vi "ABR3-Create Stimulus.vi"(0 "StimChans":T1[](xcontrol), 1 "Rep In":i32, 9 "Runtime":T26={"Ceiling"=25000.0, "Threshold"=100000.0, "Crossed?"=FALSE, "Step"=0, "Stop"=0, "Avgs"=0, "Level"=0.0, "AI Npts"=0, "Doubled?"=FALSE, "Gain"=0.0, "NWindowPts"=0, "dt"=0.0, "Cal"=path "", "Freq"=0.0, "AO Channels"=[], "AltPol"=FALSE, "AO Npts"=0, "AO Fs"=0.0, "Start"=0, "Stop max"=0, "Ear"=enum."Right", "Waveform"=enum."TONE PIP", "RepRate"=0.0, "CAP or ABR"=1, "LMasker"=0.0, "SeqVar"=enum."Signal Level", "Reps/buffer"=0, "Avg Mode"=enum."Neural/CM", "Wav"=path "", "Order"=enum."Sequential", "Levels"=[], "ControlVal"=0.0, "innerIndex"=0, "indexStep"=0} {"CAP or ABR" items=["CAP", "ABR"]}, 11 "error in (no error)":errorcluster) -> (3 "Rep Out":i32, 4 "StimChans out":T1[](xcontrol), 15 "error out":errorcluster)   [LabVIEW 2020]
uses:
  epl-vi-lib/Signal Synthesis VIs/Controls/Multichannel (Full)/Multichannel (Full).xctl
  TypeDefs/ABR3-Runtime Data.ctl
  epl-vi-lib/Utility VIs/Type Defs/Left-Right ring.ctl
  TypeDefs/ABR-Waveform Enum.ctl
  TypeDefs/ABR3-Seq Var Enum.ctl
  epl-vi-lib/Utility VIs/Array Manipulation VIs/Array-Dimensions (2D).vi
panel:
  out "Elapsed time (ms)":u32
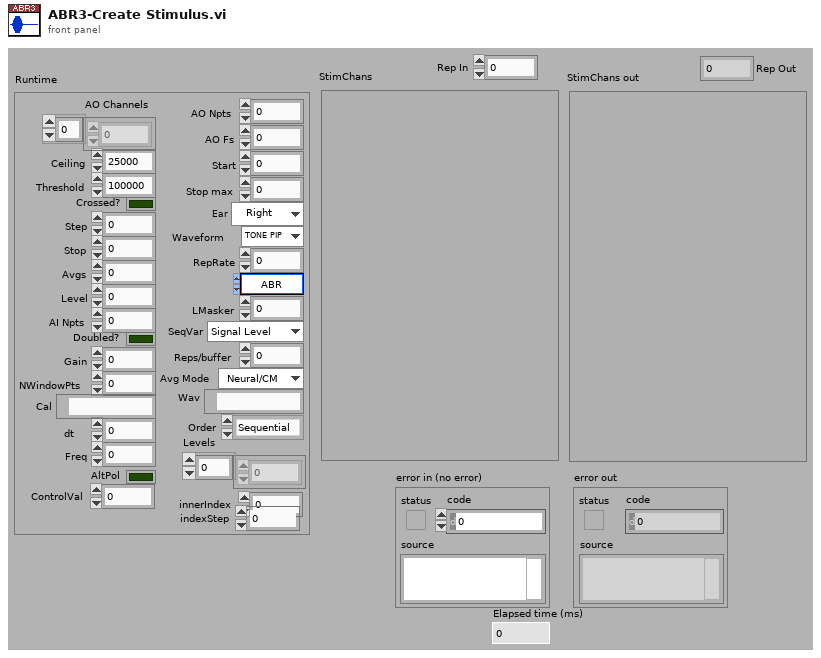
[diagram p1: front panel]
types:
  T1 = typedef "Stimulus Channel (Full).xctl/Full Stimulus Channel Data.ctl" = cluster{"Waveform":T2, "Filter":T19, "Burst":T21, "Level":T22, "Name":string, "Advanced":T24, "SAM":T25}
  T2 = typedef "Waveform XCtl.xctl/Waveform Data.ctl" = cluster{"Type":T3, "Tone":T4, "Pulse Train":T5, "Noise":T8, "File":T9, "FMSweep":T10, "Chirp Train":T11, "Complex Tone":cluster{"Params":T13, "Data":T15}, "Moving Ripple":T16}
  T3 = typedef "Waveform Enum.ctl" = enum16{"OFF", "Tone", "Noise", "Pulse Train", "File", "FM Sweep", "Chirp Train", "Complex Tone", "FM Tone", "Moving Ripple"}
  T4 = typedef "Tone Params.ctl" = cluster{"Frequency (kHz)":dbl, "Last Freq":dbl, "Last Phase":dbl}
  T5 = typedef "Pulse Train Params.ctl" = cluster{"Pulse width (us)":dbl, "Pulse rate (Hz)":dbl, "Gap (ms)":dbl, "Polarity":T6, "PT State":T7, "Asynch":bool}
  T6 = typedef "Pulse Polarity.ctl" = enum16{"POS", "NEG", "POS-NEG", "NEG-POS"}
  T7 = typedef "PT-Continuous State.ctl" = cluster{"Template":dbl[], "Nperiod":i32, "Index":i32, "Pulse Rate (Hz)":dbl, "Phase (cycles)":dbl, "Noff":i32}
  T8 = typedef "Noise Params.ctl" = cluster{"InvFilt":bool, "Noise":dbl[], "CurPt":i32, "Aweight":bool, "Seed":i32, "afile":path}
  T9 = typedef "StimFile-Params.ctl" = cluster{"Filename":path, "Signal":dbl[], "Channel":i32, "stream":bool, "offset":i32, "nreps":i32, "loops":i32, "Randomize":bool, "order":i32[], "Seed":i32, "Tokens":i32}
  T10 = typedef "FM Sweep Params.ctl" = cluster{"Rate (oct/s)":dbl, "Fmin (Hz)":dbl, "Fmax (Hz)":dbl, "Ramp (ms)":dbl, "Linear":bool}
  T11 = typedef "Chirp Train.ctl" = cluster{"Params":T12, "Data":cluster{"WF":dbl[]}}
  T12 = typedef "Chirp Train Params.ctl" = cluster{"Fmin (kHz)":dbl, "Fmax (kHz)":dbl, "Compensate":bool, "Duration (ms)":dbl}
  T13 = typedef "CT-Params.ctl" = cluster{"F0 (Hz)":dbl, "Band":cluster{"Flow (Hz)":dbl, "Fhigh (Hz)":dbl}, "Phase":T14, "Min F0 (Hz)":dbl, "Max F0 (Hz)":dbl, "ContinRandPhase":bool, "Max peak factor":dbl, "Max mod depth":dbl, "MinHarmNum":i32, "MaxHarmNum":i32, "Level Mode":enum16{"per component", "overall rms"}, "% jitter":dbl}
  T14 = typedef "CT-Phase Enum.ctl" = enum16{"Cosine", "Random", "Alternating"}
  T15 = typedef "CT-Runtime Data.ctl" = cluster{"Ncomp":i32, "MinHarm":i32, "Phase":dbl[], "Amplitude":dbl[], "Npts/frame":i32, "Last F0":dbl, "Fmin":dbl, "Fmax":dbl, "Lslope":dbl, "randphase":bool, "overall rms":bool, "fmult":dbl[], "jittered":bool}
  T16 = typedef "Moving Ripple.ctl" = cluster{"Params":T17, "Data":T18}
  T17 = typedef "Moving Ripple.Params.ctl" = cluster{"Fmin":dbl, "Fmax":dbl, "Density":dbl, "Velocity":dbl, "Depth":dbl, "Phase":dbl, "Comp/oct":i32}
  T18 = typedef "Moving Ripple.Data.ctl" = cluster{"Freq":dbl[], "A":dbl[], "phase":dbl[], "Phase":dbl}
  T19 = typedef "Advanced Filter XCtl.xctl/Filter Data.ctl" = cluster{"Type":enum16{"Lowpass", "Highpass", "Bandpass", "Bandstop", "OFF"}, "CF (kHz)":dbl, "BW (kHz)":dbl, "Cascade":bool, "Quadrature":bool, "Scale Factor":dbl, "Stages":cluster{"IIR Filter":cluster{"filter structure":enum32{"IIR 2nd Order", "IIR 4th Order"}, "Reverse Coefficients":dbl[], "Forward Coefficients":dbl[]}, "State":dbl[]}[], "Class":enum16{"Elliptic", "Butterworth"}, "Order":i32, "BWUnits":T20}
  T20 = typedef "Filter-Bandwidth Units.ctl" = enum16{"Linear", "Octaves", "Min-Max"}
  T21 = typedef "Burst Control.xctl/Burst Data.ctl" = cluster{"Active":bool, "Delay (ms)":dbl, "Duration (ms)":dbl, "Ramp (ms)":dbl, "Rate (Hz)":dbl, "Trepeat (ms)":dbl, "Repeat":bool}
  T22 = typedef "Level XCtl.xctl/Level Data.ctl" = cluster{"Level":dbl, "Units":T23, "Max":dbl, "Multiplier":dbl, "Cal File":path, "Cal":cluster{"Freq (Hz)":dbl[], "Mag (dB SPL)":dbl[], "Phase (deg)":dbl[]}}
  T23 = typedef "Level Units.ctl" = enum16{"dB atten", "dB SPL", "dB re 1 Vrms", "dB V/Hz½", "mW", "dB HL", "Volts", "dB mW"}
  T24 = typedef "Advanced Stimulus Options.xctl/Advanced Stimulus Options.ctl" = cluster{"Rep Mask":string, "AltPol":bool, "Var":string, "Expr":string, "Persist":bool}
  T25 = typedef "SAM Params.ctl" = cluster{"Active":bool, "Frequency (Hz)":dbl, "Depth":dbl, "Init Phase (cycles)":dbl, "phase (degrees)":dbl, "Asynch":bool}
  T26 = typedef "ABR3-Runtime Data.ctl" = cluster{"Ceiling":dbl, "Threshold":dbl, "Crossed?":bool, "Step":i32, "Stop":i32, "Avgs":i32, "Level":dbl, "AI Npts":i32, "Doubled?":bool, "Gain":dbl, "NWindowPts":i32, "dt":dbl, "Cal":path, "Freq":dbl, "AO Channels":i32[], "AltPol":bool, "AO Npts":i32, "AO Fs":dbl, "Start":i32, "Stop max":i32, "Ear":T27, "Waveform":T28, "RepRate":dbl, "CAP or ABR":u16, "LMasker":dbl, "SeqVar":T29, "Reps/buffer":i32, "Avg Mode":enum16{"Neural/CM", "ANOW"}, "Wav":path, "Order":enum16{"Sequential", "Random"}, "Levels":dbl[], "ControlVal":dbl, "innerIndex":i32, "indexStep":i32}
  T27 = typedef "Left-Right ring.ctl" = enum16{"Right", "Left"}
  T28 = typedef "ABR-Waveform Enum.ctl" = enum16{"TONE PIP", "CLICK", "FILE", "CHIRP", "NOISE", "VERHULST"}
  T29 = typedef "ABR3-Seq Var Enum.ctl" = enum16{"Signal Level", "Masker Level"}
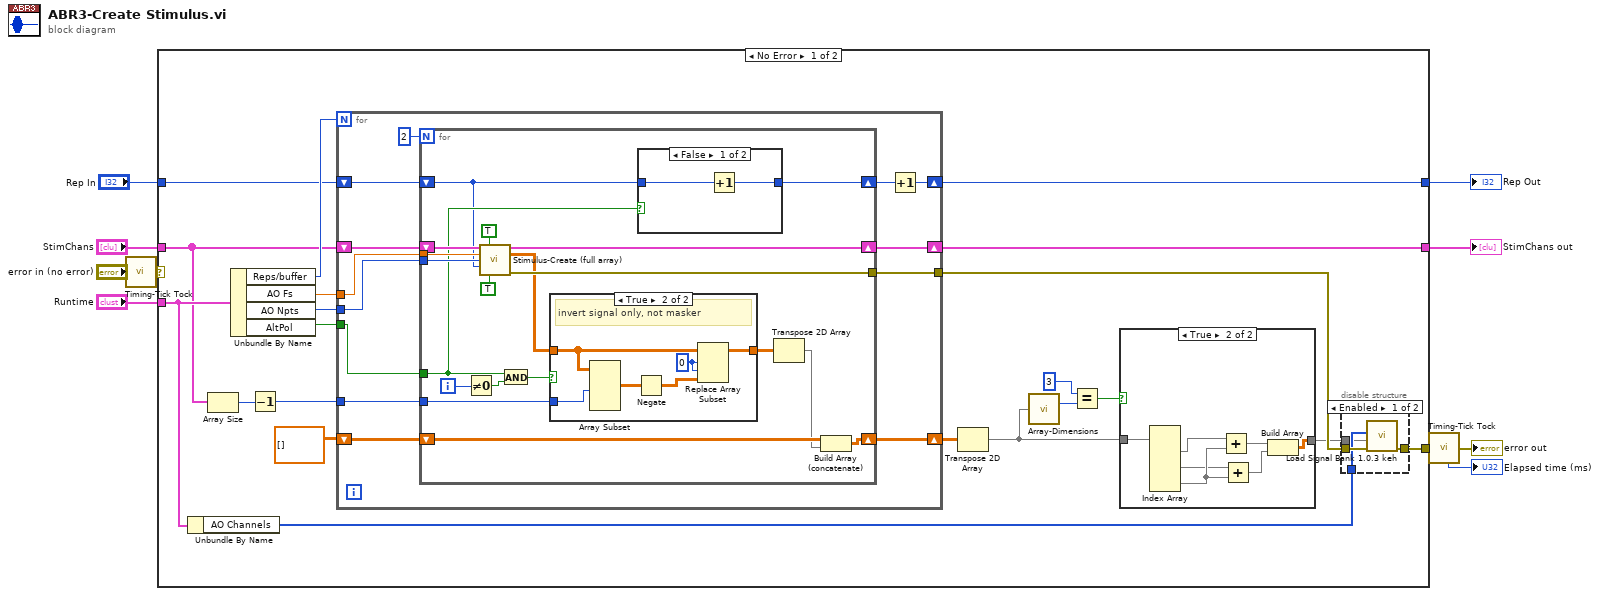
[diagram p0: block diagram]
diagram:
  n1 = call "Timing-Tick Tock.vi"("error in (no error)"="error in (no error)") -> ("error out"=w7:errorcluster)  [unwired: 5 in, 1 out]
  n2 = case shown="No Error" w7 {
    selector: w7 -> [_ w86]
    tunnel: [w25 w86] -> w10
    tunnel: "StimChans" -> [w21 _]
    tunnel: "Runtime" -> [w24 _]
    tunnel: [w30 _] -> w4
    tunnel: "Rep In" -> [w12 _]
    tunnel: [w11 _] -> w1
    frame No Error {
      n3 = Unbundle By Name(w24) -> ("AO Channels"=w23:i32[])
      n4 = Array Size(array=w21) -> (size(s)=w20:i32)
      n5 = Unbundle By Name(w24) -> ("Reps/buffer"=w22:i32, "AO Fs"=w31:dbl, "AO Npts"=w29:i32, "AltPol"=w28:bool)
      n6 = Decrement(x=w20) -> (x-1=w19:i32)
      n7 = for {
        N: w22 -> [_]
        tunnel: w31 -> [w56]
        tunnel: w29 -> [w54]
        tunnel: w28 -> [w53]
        tunnel: [w50] -> w26
        shift-right: [w55] -> w30
        shift-left: w21 -> [w49]
        shift-right: [w51] -> w14
        shift-left: dbl[][] [] -> [w52]
        tunnel: w19 -> [w47]
        shift-right: [w44] -> w11
        shift-left: w12 -> [w46]
        n8 = for {
          N: 2 -> [_]
          tunnel: w56 -> [w75]
          tunnel: [w74] -> w50
          tunnel: w54 -> [w73]
          tunnel: w53 -> [w59]
          shift-right: [w61] -> w51
          shift-left: w52 -> [w63]
          shift-right: [w64] -> w55
          shift-left: w49 -> [w65]
          tunnel: w47 -> [w60]
          shift-right: [w58] -> w45
          shift-left: w46 -> [w57]
          i -> [w66]
          n9 = Not Equal To 0?(x=w66) -> (x != 0?=w67:bool)
          n10 = call "Stimulus-Create (full array).vi"("StimChan"=w65, "Apply multipliers? (F)"=TRUE, "Sampling Rate (Hz)"=w75, "Npts"=w73, "Rep Num"=w57, "Zero unused (F)"=TRUE) -> ("StimChan Out"=w64:T1[], "Waveform"=w70:dbl[][], "error out"=w74:errorcluster)  [unwired: 6 in, 1 out]
          n11 = And(x=w59, y=w67) -> (x .and. y?=w68:bool)
          n12 = case shown="True" w68 {
            tunnel: w70 -> [w79 w84]
            tunnel: [w79 w81] -> w69
            tunnel: w60 -> [_ w80]
            frame False {
            }
            frame True {
              w82 = 0 ("index (row)")
              # "invert signal only, not masker"
              n13 = Array Subset(array=w84, length (row)=w80) -> (w85:dbl[][])  [unwired: 3 in]
              n14 = Negate(x=w85) -> (-x=w83:dbl[][])
              n15 = Replace Array Subset(array=w84, new element=w83, index (row)=w82, index (col)=w82) -> (w81:dbl[][])
            }
          }
          n16 = case shown="False" w59 {
            tunnel: w57 -> [w77 w78]
            tunnel: [w76 w78] -> w58
            frame False {
              n17 = Increment(x=w77) -> (x+1=w76:i32)
            }
            frame True {
            }
          }
          n18 = Transpose 2D Array(2D array=w69) -> (transposed array=w62:dbl[][])
          n19 = Build Array (concatenate)(w63, w62) -> (w61:dbl[][])
        }
        n20 = Increment(x=w45) -> (x+1=w44:i32)
      }
      n21 = Transpose 2D Array(2D array=w14) -> (transposed array=w13:dbl[][])
      n22 = call-poly "Array-Dimensions.vi"("2D Array"=w13) -> ("# rows"=w18:i32)  [unwired: 13 in, 1 out]
      n23 = Equal?(x=3, y=w18) -> (x = y?=w16:bool)
      n24 = case shown="True" w16 {
        tunnel: [w32 w33] -> w15
        tunnel: w13 -> [w32 w39]
        frame False {
        }
        frame True {
          n25 = Index Array(array=w39) -> (element #1=w38:dbl[], element #2=w36:dbl[], element #3=w37:dbl[])  [unwired: 6 in]
          n26 = Add(x=w38, y=w37) -> (x+y=w35:dbl[])
          n27 = Add(x=w36, y=w37) -> (x+y=w34:dbl[])
          n28 = Build Array(w35, w34) -> (w33:dbl[][])
        }
      }
      n29 = disable-structure shown="Enabled" {
        disable-tunnel: w26 -> [w43 _]
        disable-tunnel: [w42 _] -> w25
        disable-tunnel: w23 -> [w41 _]
        disable-tunnel: w15 -> [w40 _]
        frame Enabled {
          n30 = call "Load Signal Bank 1.0.3 keh.vi"("error in (no error)"=w43, "Input array"=w40, "Active AO Array"=w41) -> ("error out"=w42:errorcluster)  [unwired: 6 in, 2 out]
        }
        frame Disabled {
        }
      }
    }
    frame Error {
    }
  }
  "StimChans out" <- w4
  "Rep Out" <- w1
  n31 = call "Timing-Tick Tock.vi"("error in (no error)"=w10) -> ("Elapsed time (ms)"=→"Elapsed time (ms)":u32, "error out"=→"error out":errorcluster)  [unwired: 5 in]
